vi "dfd_Set Filter Modeling.vi"(5 "output integer word length":T1, 6 "output round-off mode":T2, 7 "input iwl (1)":i16=1, 8 "error in (no error)":errorcluster, 9 "output wl (16)":i16=16, 10 "input wl (16)":i16=16, 11 "filter in":T3={"mSRate_Fs"=1.0, "mSRate_Version"="1.0", "mSRate_Comments"="", "mSRate_OrgCoef"={"type"=enum."Undefined", "gain"=1.0, "coef a (k)"=[], "coef b (v)"=[]}, "mSRate_CurCoef"={"type"=enum."Undefined", "gain"=1.0, "coef a (k)"=[], "coef b (v)"=[]}, "mSRate_Quantized?"=FALSE, "mSRate_QCoef"={"type"=enum."Undefined", "gain"=1.0, "coef a (k)"=[], "coef b (v)"=[]}, "mSRate_QSettings"=[], "mSRate_Order"=0, "mSRate_Scaling"={"mSRate_ScaleByPowerOf2?"=FALSE, "mSRate_ScaleType"=enum."No Norm"}} {"mSRate_QSettings"."source" items=["Coef a/k"=0, "Coef b/v"=7, "Input"=1, "Output"=2, "Multiplicand"=3, "Product"=4, "Sum"=5, "Delay"=6, "Gain"=8]}) -> (0 "error out":errorcluster, 3 "filter out":T3={"mSRate_Fs"=1.0, "mSRate_Version"="1.0", "mSRate_Comments"="", "mSRate_OrgCoef"={"type"=enum."Undefined", "gain"=1.0, "coef a (k)"=[], "coef b (v)"=[]}, "mSRate_CurCoef"={"type"=enum."Undefined", "gain"=1.0, "coef a (k)"=[], "coef b (v)"=[]}, "mSRate_Quantized?"=FALSE, "mSRate_QCoef"={"type"=enum."Undefined", "gain"=1.0, "coef a (k)"=[], "coef b (v)"=[]}, "mSRate_QSettings"=[], "mSRate_Order"=0, "mSRate_Scaling"={"mSRate_ScaleByPowerOf2?"=FALSE, "mSRate_ScaleType"=enum."No Norm"}} {"mSRate_QSettings"."source" items=["Coef a/k"=0, "Coef b/v"=7, "Input"=1, "Output"=2, "Multiplicand"=3, "Product"=4, "Sum"=5, "Delay"=6, "Gain"=8]})   [LabVIEW 2017, in "NI_DigFilter_FXP.lvlib"]
uses:
  <vilib>/addons/Digital Filter Design/NI_DigFilter_FXP.lvlib
  <vilib>/addons/Digital Filter Design/_Objects.llb/DFD Filter Obj.ctl
  <vilib>/addons/Digital Filter Design/_Objects.llb/DFD Filter Coef.ctl
  <vilib>/addons/Digital Filter Design/_Objects.llb/DFD Filter Structure Type Selector.ctl
  <vilib>/addons/Digital Filter Design/_Objects.llb/dfd_Internal Quantization Settings.ctl
  <vilib>/addons/Digital Filter Design/_Objects.llb/dfd_Internal Quantization Srcs.ctl
  <vilib>/addons/Digital Filter Design/_Objects.llb/DFD Coef Norm Type.ctl
  <vilib>/addons/Digital Filter Design/_Objects.llb/DFD Round-off Mode.ctl
  <vilib>/addons/Digital Filter Design/_Objects.llb/DFD Output Iwl Obj.ctl
  <vilib>/addons/Digital Filter Design/NI_DigFilterLicensed.lvlib
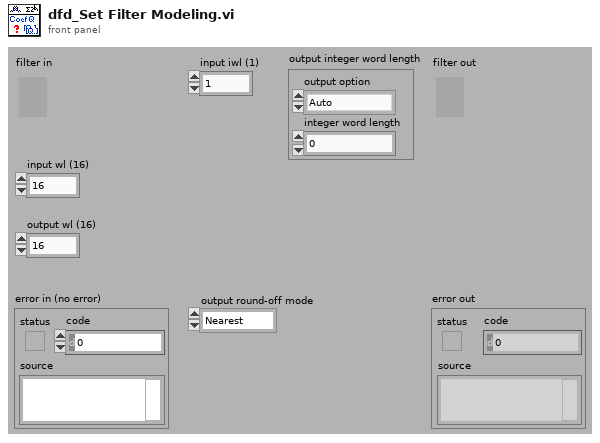
[diagram p1: front panel]
types:
  T1 = typedef "NI_DigFilterLicensed.lvlib/DFD Output Iwl Obj.ctl" = cluster{"output option":enum16{"Auto", "Same As Input", "User Defined"}, "integer word length":i16}
  T2 = typedef "NI_DigFilterLicensed.lvlib/DFD Round-off Mode.ctl" = enum16{"Nearest", "Truncation"}
  T3 = typedef "NI_DigFilterLicensed.lvlib/DFD Filter Obj.ctl" = cluster{"mSRate_Fs":dbl, "mSRate_Version":string, "mSRate_Comments":string, "mSRate_OrgCoef":T4, "mSRate_CurCoef":T4, "mSRate_Quantized?":bool, "mSRate_QCoef":T4, "mSRate_QSettings":T6[], "mSRate_Order":i32, "mSRate_Scaling":cluster{"mSRate_ScaleByPowerOf2?":bool, "mSRate_ScaleType":T8}}
  T4 = typedef "NI_DigFilterLicensed.lvlib/DFD Filter Coef.ctl" = cluster{"type":T5, "gain":dbl, "coef a (k)":dbl[], "coef b (v)":dbl[]}
  T5 = typedef "NI_DigFilterLicensed.lvlib/DFD Filter Structure Type Selector.ctl" = enum16{"Undefined", "FIR Direct Form", "FIR Direct Form Transposed", "FIR Symmetric", "FIR Antisymmetric", "IIR Direct Form I", "IIR Direct Form I Transposed", "IIR Direct Form II", "IIR Direct Form II Transposed", "IIR Cascaded Second Order Sections Form I", "IIR Cascaded Second Order Sections Form I Transposed", "IIR Cascaded Second Order Sections Form II", "IIR Cascaded Second Order Sections Form II Transposed", "Lattice Allpass (basic sections)", "Lattice Allpass (one multiplier sections)", "Lattice Allpass (normalized sections)", "Lattice AR (basic sections)", "Lattice AR (one multiplier sections)", "Lattice AR (normalized sections)", "Lattice MA (minimum phase)", "Lattice MA (maximum phase)", "Lattice ARMA (basic sections)", "Lattice ARMA (one multiplier sections)", "Lattice ARMA (normalized sections)"}
  T6 = typedef "NI_DigFilterLicensed.lvlib/dfd_Internal Quantization Settings.ctl" = cluster{"source":T7, "wl":i16, "iwl":i16, "overflow mode":enum16{"Saturation", "Wrap"}, "rounding mode":enum16{"Nearest", "Truncation"}, "signed?":bool}
  T7 = typedef "NI_DigFilterLicensed.lvlib/dfd_Internal Quantization Srcs.ctl" = u16
  T8 = typedef "NI_DigFilterLicensed.lvlib/DFD Coef Norm Type.ctl" = enum16{"No Norm", "Time Domain 1-Norm", "Time Domain 2-Norm", "Time Domain Inf-Norm"}
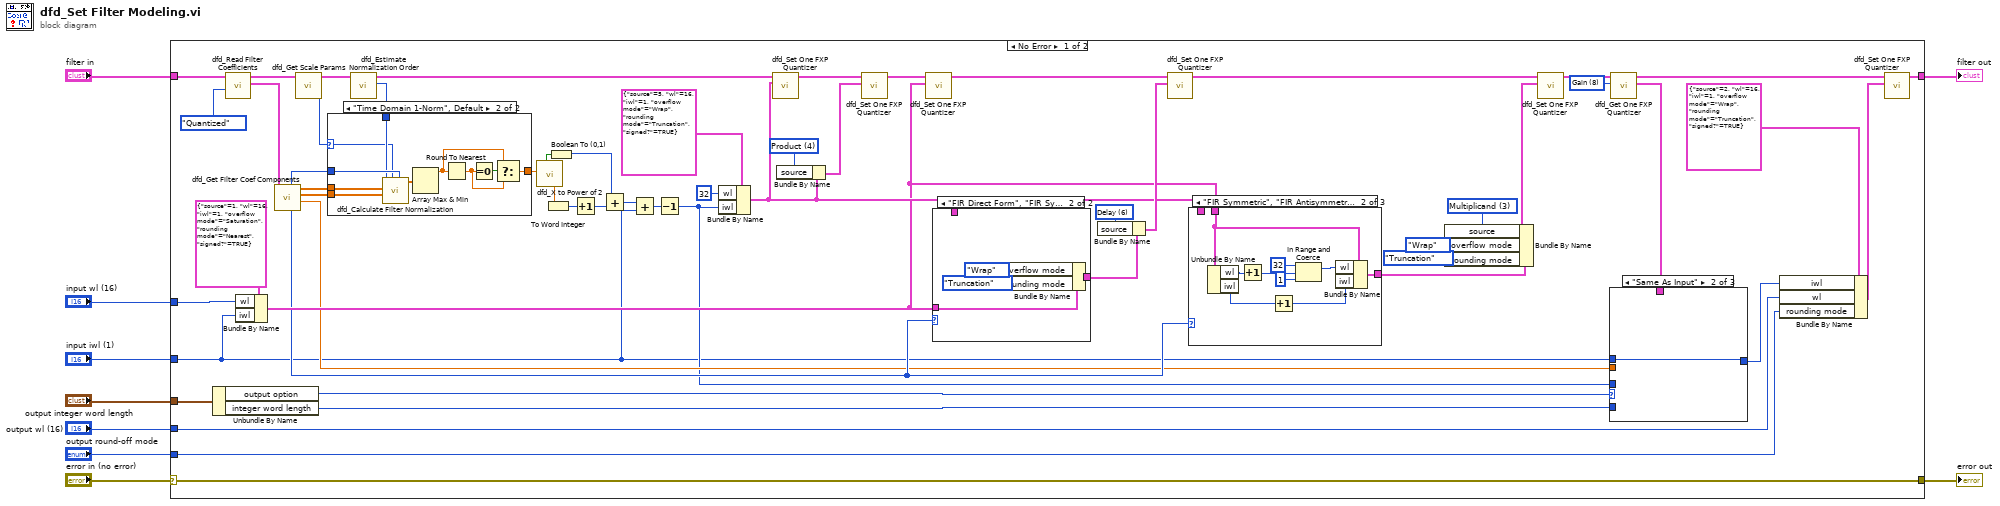
[diagram p0: block diagram]
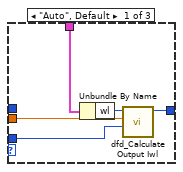
[diagram p2: hidden frame]
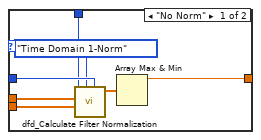
[diagram p4: hidden frame]
diagram:
  n1 = case shown="No Error" "error in (no error)" {
    selector: "error in (no error)" -> [w33 w106]
    tunnel: "filter in" -> [w63 w107]
    tunnel: "input wl (16)" -> [w60 _]
    tunnel: [w39 w107] -> w7
    tunnel: "output wl (16)" -> [w38 _]
    tunnel: "output round-off mode" -> [w36 _]
    tunnel: [w33 w106] -> w3
    tunnel: "input iwl (1)" -> [w10 _]
    tunnel: "output integer word length" -> [w13 _]
    frame No Error {
      w47 = T7 3 items=["Coef a/k"=0, "Coef b/v"=7, "Input"=1, "Output"=2, "Multiplicand"=3, "Product"=4, "Sum"=5, "Delay"=6, "Gain"=8] ("source")
      w53 = T7 8 items=["Coef a/k"=0, "Coef b/v"=7, "Input"=1, "Output"=2, "Multiplicand"=3, "Product"=4, "Sum"=5, "Delay"=6, "Gain"=8] ("quantization source")
      w57 = T7 6 items=["Coef a/k"=0, "Coef b/v"=7, "Input"=1, "Output"=2, "Multiplicand"=3, "Product"=4, "Sum"=5, "Delay"=6, "Gain"=8] ("source")
      w61 = T7 4 items=["Coef a/k"=0, "Coef b/v"=7, "Input"=1, "Output"=2, "Multiplicand"=3, "Product"=4, "Sum"=5, "Delay"=6, "Gain"=8] ("source")
      n2 = Unbundle By Name(w13) -> ("output option"=w12:enum16{"Auto", "Same As Input", "User Defined"}, "integer word length"=w11:i16)
      n3 = call <vilib>:"dfd_Read Filter Coefficients.vi"("coef source"=enum16{"Original", "Current", "Quantized"}."Quantized", "filter in"=w63) -> ("filter coef"=w65:T4, "filter out"=w32:T3)  [unwired: 1 in, 7 out]
      n4 = Bundle By Name(cluster=T6 {"source"=1, "wl"=16, "iwl"=1, "overflow mode"=enum."Saturation", "rounding mode"=enum."Nearest", "signed?"=TRUE} ("input cluster"), "wl"=w60, "iwl"=w10) -> (w43:T6)
      n5 = call <vilib>:"dfd_Get Filter Coef Components.vi"("filter coef"=w65) -> ("gain"=w26:dbl, "coef a (k)"=w27:dbl[], "coef b (v)"=w28:dbl[], "type"=w29:T5)  [unwired: 1 in, 6 out]
      n6 = call <vilib>:"dfd_Get Scale Params.vi"("filter in"=w32) -> ("scale type"=w17:T8, "dup filter"=w31:T3)  [unwired: 9 out]
      n7 = call <vilib>:"dfd_Estimate Normalization Order.vi"("filter in"=w31) -> ("iteration"=w21:i32, "filter out"=w30:T3)  [unwired: 1 in, 8 out]
      n8 = case shown="\"Time Domain 1-Norm\", Default" w17 {
        selector: w17 -> [_ w84]
        tunnel: w29 -> [w79 w89]
        tunnel: w28 -> [w78 w88]
        tunnel: w27 -> [w77 w87]
        tunnel: [w75 w82] -> w24
        tunnel: w21 -> [w74 w85]
        frame "No Norm" {
          n9 = call <vilib>:"dfd_Calculate Filter Normalization.vi"("structure type"=w79, "scale type"=DFD_Coef_Norm_Type."Time Domain 1-Norm", "coefficients a/k"=w77, "coefficients b/v"=w78, "iterations"=w74) -> ("norm"=w76:dbl[])  [unwired: 1 in, 5 out]
          n10 = Array Max & Min(array=w76) -> (max value=w75:dbl)  [unwired: 3 out]
        }
        frame "Time Domain 1-Norm", Default {
          n11 = call <vilib>:"dfd_Calculate Filter Normalization.vi"("structure type"=w89, "scale type"=w84, "coefficients a/k"=w87, "coefficients b/v"=w88, "iterations"=w85) -> ("norm"=w86:dbl[])  [unwired: 1 in, 5 out]
          n12 = Array Max & Min(array=w86) -> (max value=w81:dbl)  [unwired: 3 out]
          n13 = Round To Nearest(number=w81) -> (nearest integer value=w80:dbl)
          n14 = Equal To 0?(x=w80) -> (x = 0?=w83:bool)
          n15 = Select(t=w81, s=w83, f=w80) -> (s? t:f=w82:dbl)
        }
      }
      n16 = call <vilib>:"dfd_X to Power of 2.vi"("x"=w24) -> ("n"=w22:dbl, "is 2^n?"=w20:bool)  [unwired: 9 out]
      n17 = To Word Integer(number=w22) -> (16bit integer=w23:i16)
      n18 = Boolean To (0,1)(Boolean=w20) -> (0, 1=w18:i16)
      n19 = Increment(x=w23) -> (x+1=w19:i16)
      n20 = Add(x=w18, y=w19) -> (x+y=w16:i16)
      n21 = Add(x=w16, y=w10) -> (x+y=w15:i16)
      n22 = Decrement(x=w15) -> (x-1=w14:i16)
      n23 = Bundle By Name(cluster=T6 {"source"=5, "wl"=16, "iwl"=1, "overflow mode"=enum."Wrap", "rounding mode"=enum."Truncation", "signed?"=TRUE} ("input cluster"), "wl"=i16 32, "iwl"=w14) -> (w44:T6)
      n24 = call <vilib>:"dfd_Set One FXP Quantizer.vi"("quantization settings"=w44, "filter in"=w30) -> ("filter out"=w59:T3)  [unwired: 1 in, 8 out]
      n25 = Bundle By Name(cluster=w44, "source"=w61) -> (w45:T6)
      n26 = call <vilib>:"dfd_Set One FXP Quantizer.vi"("quantization settings"=w45, "filter in"=w59) -> ("filter out"=w58:T3)  [unwired: 1 in, 8 out]
      n27 = call <vilib>:"dfd_Set One FXP Quantizer.vi"("quantization settings"=w43, "filter in"=w58) -> ("filter out"=w54:T3)  [unwired: 1 in, 8 out]
      n28 = case shown="\"FIR Direct Form\", \"FIR Symmetric\", \"FIR Antisymmetric\"" w29 {
        tunnel: w43 -> [_ w102]
        tunnel: [w101 w103] -> w56
        tunnel: w44 -> [w101 _]
        frame "Undefined", Default {
        }
        frame "FIR Direct Form", "FIR Symmetric", "FIR Antisymmetric" {
          n29 = Bundle By Name(cluster=w102, "overflow mode"=enum16{"Saturation", "Wrap"}."Wrap" ("o_mode"), "rounding mode"=enum16{"Nearest", "Truncation"}."Truncation" ("q_mode")) -> (w103:T6)
        }
      }
      n30 = Bundle By Name(cluster=w56, "source"=w57) -> (w55:T6)
      n31 = call <vilib>:"dfd_Set One FXP Quantizer.vi"("quantization settings"=w55, "filter in"=w54) -> ("filter out"=w41:T3)  [unwired: 1 in, 8 out]
      n32 = case shown="\"FIR Symmetric\", \"FIR Antisymmetric\"" w29 {
        tunnel: w44 -> [w90 _ _]
        tunnel: [w90 w99 w100] -> w42
        tunnel: w43 -> [_ w98 w100]
        frame "Undefined", Default {
        }
        frame "FIR Symmetric", "FIR Antisymmetric" {
          n33 = Unbundle By Name(w98) -> ("wl"=w96:i16, "iwl"=w92:i16)
          n34 = Increment(x=w96) -> (x+1=w95:i16)
          n35 = Increment(x=w92) -> (x+1=w97:i16)
          n36 = In Range and Coerce(upper limit=i16 32, x=w95, lower limit=i16 1) -> (coerced(x)=w91:i16)  [unwired: 1 out]
          n37 = Bundle By Name(cluster=w98, "wl"=w91, "iwl"=w97) -> (w99:T6)
        }
        frame "FIR Direct Form", "FIR Direct Form Transposed" {
        }
      }
      n38 = Bundle By Name(cluster=w42, "source"=w47, "overflow mode"=enum16{"Saturation", "Wrap"}."Wrap" ("o_mode"), "rounding mode"=enum16{"Nearest", "Truncation"}."Truncation" ("q_mode")) -> (w46:T6)
      n39 = call <vilib>:"dfd_Set One FXP Quantizer.vi"("quantization settings"=w46, "filter in"=w41) -> ("filter out"=w40:T3)  [unwired: 1 in, 8 out]
      n40 = call <vilib>:"dfd_Get One FXP Quantizer.vi"("quantization source"=w53, "filter in"=w40) -> ("quantization settings"=w52:T6, "filter out"=w50:T3)  [unwired: 1 in, 7 out]
      n41 = case shown="\"Same As Input\"" w12 {
        tunnel: w52 -> [w70 _ _]
        tunnel: w26 -> [w69 _ _]
        tunnel: [w67 w71 w72] -> w25
        tunnel: w14 -> [w66 _ _]
        tunnel: w11 -> [_ _ w72]
        tunnel: w10 -> [_ w71 _]
        frame "Auto", Default {
          n42 = Unbundle By Name(w70) -> ("wl"=w68:i16)
          n43 = call <vilib>:"dfd_Calculate Output Iwl.vi"("sum iwl"=w66, "gain value"=w69, "gain wl"=w68) -> ("output iwl"=w67:i16)  [unwired: 8 out]
        }
        frame "Same As Input" {
        }
        frame "User Defined" {
        }
      }
      n44 = Bundle By Name(cluster=T6 {"source"=2, "wl"=16, "iwl"=1, "overflow mode"=enum."Wrap", "rounding mode"=enum."Truncation", "signed?"=TRUE} ("input cluster"), "iwl"=w25, "wl"=w38, "rounding mode"=w36) -> (w37:T6)
      n45 = call <vilib>:"dfd_Set One FXP Quantizer.vi"("quantization settings"=w37, "filter in"=w50) -> ("filter out"=w39:T3)  [unwired: 1 in, 8 out]
    }
    frame Error {
    }
  }
  "filter out" <- w7
  "error out" <- w3
